vi "Teardown.vi"(8 "error in (no error)":errorcluster, 11 "LUnit Error Handler Tests In":refnum<class "Error Handler Tests.lvclass">) -> (0 "error out":errorcluster, 3 "LUnit Error Handler Tests Out":refnum<class "Error Handler Tests.lvclass">)   [LabVIEW 2020, in "Error Handler Tests.lvclass"]
uses:
  Error Handler Tests.lvclass
  Error Handler Tests.lvclass/Error Handler Tests.ctl
  source/User Interface/Support/Paths.lvlib
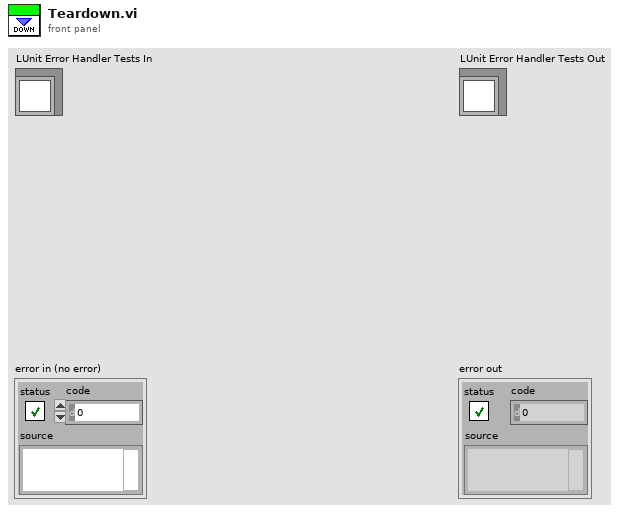
[diagram p1: front panel]
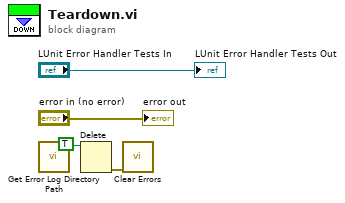
[diagram p0: block diagram]
diagram:
  n1 = call "Get Error Log Directory Path.vi"() -> ("Error Log Path"=w3:path)  [unwired: 11 in]
  n2 = Delete(path (use dialog)=w3, entire hierarchy (F)=TRUE) -> (error out=w2:errorcluster)  [unwired: 3 in, 2 out]
  n3 = call <vilib>:"Clear Errors.vi"("error in (no error)"=w2) -> ()  [unwired: 5 in, 2 out]
  "error out" <- "error in (no error)"
  "LUnit Error Handler Tests Out" <- "LUnit Error Handler Tests In"
